vi "Differential_Drive_Kinematics_Curvature_Control_Curvature_In.vi"(8 "Scale_Down_For_Turn":bool, 9 "curvature(in^-1)":dbl=0.06667, 10 "Linear_Throttle":dbl) -> (1 "Right_Motor_Velocity(rotations/s)":dbl, 2 "Left_Motor_Velocity(rotations/s)":dbl)   [LabVIEW 2019]
panel:
  in  "Gear_Reduction(output/input)":dbl=1.0
  in  "Wheel_Base_Radius(in)":dbl=11.87
  in  "Wheel_Radius(in)":dbl=3.0
  in  "Max_Linear_Speed(in/s)":dbl=170.0
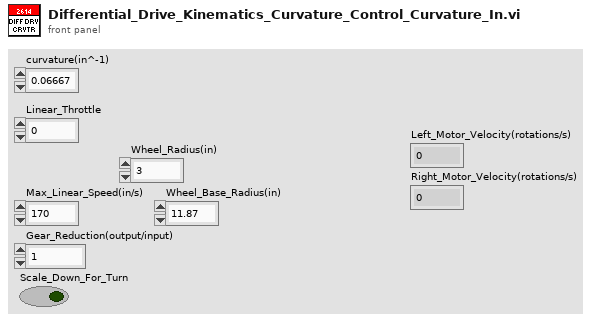
[diagram p1: front panel]
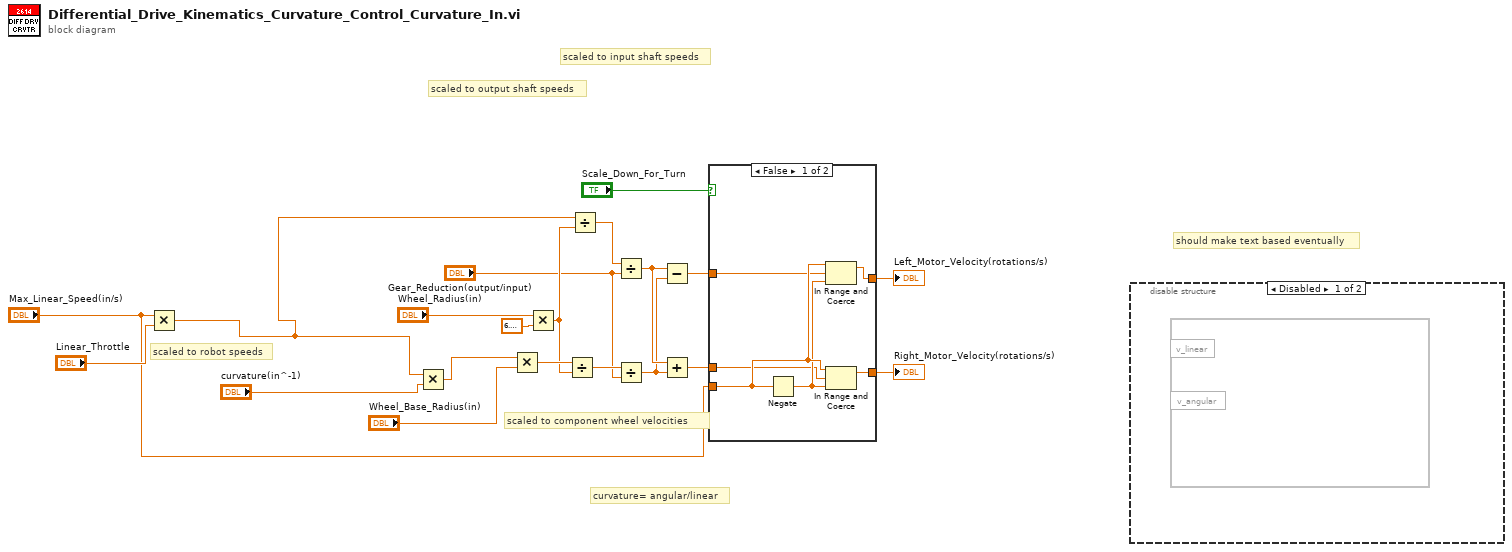
[diagram p0: block diagram]
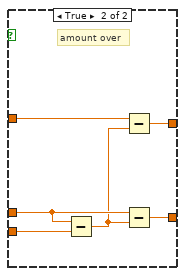
[diagram p3: hidden frame]
diagram:
  # "curvature= angular/linear"
  # "should make text based eventually"
  # "scaled to component wheel velocities"
  # "scaled to input shaft speeds"
  # "scaled to output shaft speeds"
  # "scaled to robot speeds"
  n1 = Multiply(x="Max_Linear_Speed(in/s)", y="Linear_Throttle") -> (x*y=w2:dbl)
  n2 = Multiply(x=w2, y="curvature(in^-1)") -> (x*y=w3:dbl)
  n3 = Multiply(x=w3, y="Wheel_Base_Radius(in)") -> (x*y=w15:dbl)
  n4 = Multiply(x="Wheel_Radius(in)", y=6.283185307179586) -> (x*y=w14:dbl)
  n5 = Divide(x=w15, y=w14) -> (x/y=w13:dbl)
  n6 = Divide(x=w2, y=w14) -> (x/y=w17:dbl)
  n7 = Divide(x=w17, y="Gear_Reduction(output/input)") -> (x/y=w11:dbl)
  n8 = Divide(x=w13, y="Gear_Reduction(output/input)") -> (x/y=w10:dbl)
  n9 = Subtract(x=w11, y=w10) -> (x-y=w7:dbl)
  n10 = Add(x=w11, y=w10) -> (x+y=w6:dbl)
  n11 = case shown="False" "Scale_Down_For_Turn" {
    tunnel: "Max_Linear_Speed(in/s)" -> [w26 w32]
    tunnel: w7 -> [w24 w29]
    tunnel: w6 -> [w23 w30]
    tunnel: [w22 w31] -> w5
    tunnel: [w21 w27] -> w4
    frame False {
      n12 = Negate(x=w26) -> (-x=w25:dbl)
      n13 = In Range and Coerce(upper limit=w26, x=w24, lower limit=w25) -> (coerced(x)=w21:dbl)  [unwired: 1 out]
      n14 = In Range and Coerce(upper limit=w26, x=w23, lower limit=w25) -> (coerced(x)=w22:dbl)  [unwired: 1 out]
    }
    frame True {
      # "amount over"
      n15 = Subtract(x=w30, y=w32) -> (x-y=w28:dbl)
      n16 = Subtract(x=w29, y=w28) -> (x-y=w27:dbl)
      n17 = Subtract(x=w30, y=w28) -> (x-y=w31:dbl)
    }
  }
  "Right_Motor_Velocity(rotations/s)" <- w5
  "Left_Motor_Velocity(rotations/s)" <- w4
  n18 = disable-structure shown="Disabled" {
    frame Disabled {
      n19 = formula code=""() -> ()  [unwired: 2 in]
    }
    frame Enabled {
    }
  }
